vi "范围随机数.vi"(1 "MIN(0)":dbl, 2 "MAX(10)":dbl) -> (0 "OUT":dbl format="%#.6g")   [LabVIEW 2018]
panel:
  # "取得指定范围的随机数"
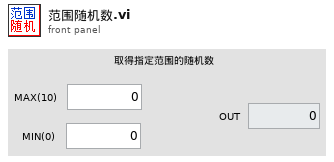
[diagram p1: front panel]
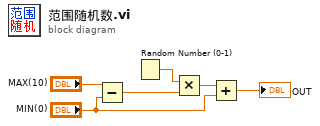
[diagram p0: block diagram]
diagram:
  n1 = Subtract(x="MAX(10)", y="MIN(0)") -> (x-y=w1:dbl)
  n2 = Random Number (0-1)() -> (number: 0 to 1=w5:dbl)
  n3 = Multiply(x=w5, y=w1) -> (x*y=w4:dbl)
  n4 = Add(x=w4, y="MIN(0)") -> (x+y=→"OUT":dbl)
